vi "Write Dictionary Element.vi"(8 "error in (no error)":errorcluster, 9 "value":variant, 10 "key":string, 11 "Control Experiment in":refnum<class "Control Experiment.lvclass">) -> (0 "error out":errorcluster, 3 "Control Experiment out":refnum<class "Control Experiment.lvclass">)   [LabVIEW 2019, in "Control Experiment.lvclass"]
uses:
  Control Experiment.lvclass
  <userlib>/LevyLab/LV-Data/LV-Data/Typedefs/Dictionary--cluster.ctl
  Control Experiment.lvclass/Control Experiment.ctl
  <userlib>/_OpenG.lib/dictionary/dictionary.llb/Dictionary Update (by scalar value)__ogtk.vi
  <userlib>/LevyLab/LV-Data/LV-Data/LV-Data.lvclass
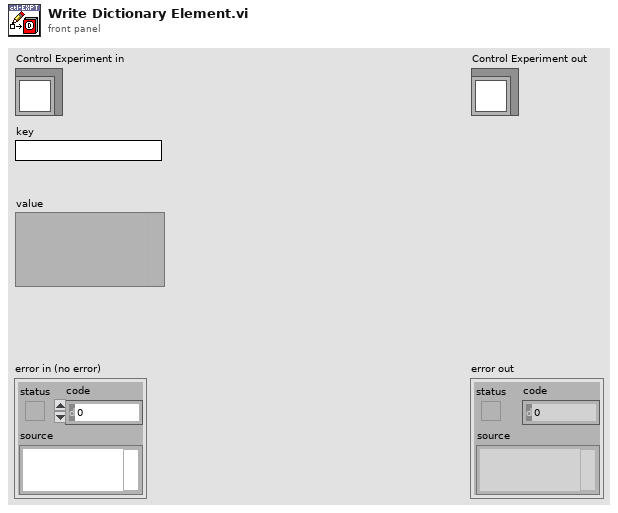
[diagram p1: front panel]
types:
  T1 = typedef "LV-Data.lvclass/Dictionary--cluster.ctl" = cluster{"key":string, "value":variant}
  T2 = typedef "Dictionary Object RefNum__ogtk.ctl" = refnum<k1>
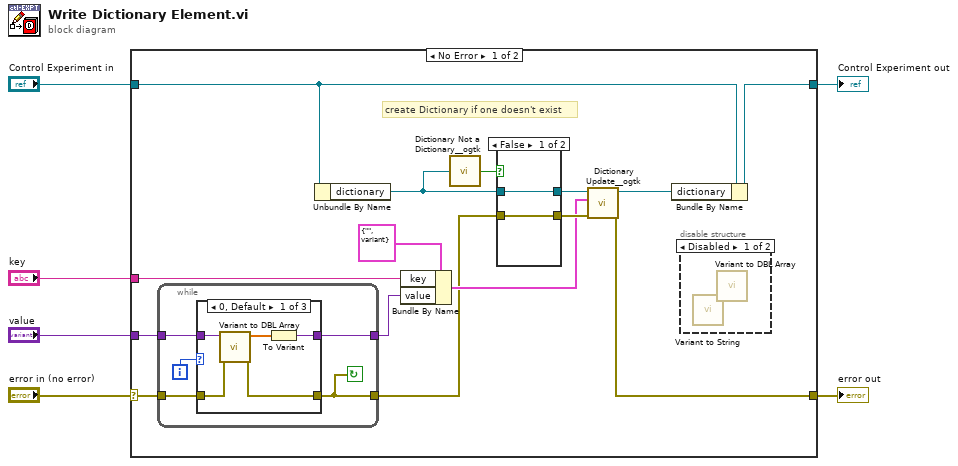
[diagram p0: block diagram]
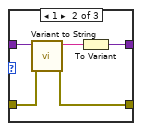
[diagram p2: hidden frame]
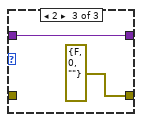
[diagram p3: hidden frame]
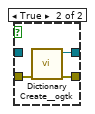
[diagram p5: hidden frame]
diagram:
  n1 = case shown="No Error" "error in (no error)" {
    selector: "error in (no error)" -> [w11 w44]
    tunnel: [w17 w44] -> w5
    tunnel: [w21 w45] -> w3
    tunnel: "Control Experiment in" -> [w19 w45]
    tunnel: "key" -> [w20 _]
    tunnel: "value" -> [w12 _]
    frame No Error {
      # "create Dictionary if one doesn't exist"
      n2 = while {
        tunnel: w12 -> [w26]
        tunnel: [w25] -> w7
        tunnel: w11 -> [w24]
        tunnel: [w23] -> w10
        i -> [w22]
        stop <- w23 continue-if-true
        n3 = case shown="0, Default" w22 {
          tunnel: w26 -> [w31 w36 w37]
          tunnel: [w27 w32 w37] -> w25
          tunnel: w24 -> [w29 w34 _]
          tunnel: [w28 w33 errorcluster {"status"=FALSE, "code"=0, "source"=""} ("error out")] -> w23
          frame 0, Default {
            n4 = call <userlib>:"Variant to DBL Array.vi"("error in (no error)"=w29, "Data (Variant)"=w31) -> ("error out"=w28:errorcluster, "1D Array"=w30:dbl[])  [unwired: 7 in, 1 out]
            n5 = To Variant(anything=w30) -> (Variant=w27:variant)
          }
          frame 1 {
            n6 = call <userlib>:"Variant to String.vi"("error in (no error)"=w34, "Data (Variant)"=w36) -> ("error out"=w33:errorcluster, "String"=w35:string)  [unwired: 8 in]
            n7 = To Variant(anything=w35) -> (Variant=w32:variant)
          }
          frame 2 {
          }
        }
      }
      n8 = Unbundle By Name(w19) -> ("dictionary"=w9:T2)
      n9 = Bundle By Name(cluster=T1 {"key"="", "value"=variant} ("key-value"), "key"=w20, "value"=w7) -> (w13:T1)
      n10 = call <userlib>:"Dictionary Not a Dictionary__ogtk.vi"("dictionary"=w9) -> ("not a dictionary?"=w15:bool)
      n11 = case shown="False" w15 {
        tunnel: [w40 w43] -> w16
        tunnel: w9 -> [w40 _]
        tunnel: [w39 w42] -> w14
        tunnel: w10 -> [w39 w41]
        frame False {
        }
        frame True {
          n12 = call <userlib>:"Dictionary Create__ogtk.vi"("error in (no error)"=w41) -> ("error out"=w42:errorcluster, "dictionary out"=w43:T2)  [unwired: 9 in]
        }
      }
      n13 = call-poly <userlib>:"Dictionary Update__ogtk.vi"("error in (no error)"=w14, "key-value"=w13, "dictionary"=w16) -> ("error out"=w17:errorcluster, "dictionary out"=w18:T2)  [unwired: 6 in, 1 out]
      n14 = Bundle By Name(cluster=w19, "dictionary"=w18) -> (w21:refnum<class "Control Experiment.lvclass">)
      n15 = disable-structure shown="Disabled" {
        frame Disabled {
          n16 = call <userlib>:"Variant to String.vi"() -> ()  [unwired: 10 in, 2 out]
          n17 = call <userlib>:"Variant to DBL Array.vi"() -> ()  [unwired: 10 in, 2 out]
        }
        frame Enabled {
        }
      }
    }
    frame Error {
    }
  }
  "error out" <- w5
  "Control Experiment out" <- w3
